vi "NegativeImage.vi"(11 "Picture in":picture) -> (3 "New Picture out":picture)   [LabVIEW 2023]
doc: "This VI creates a negative of the input picture. \n\nPicture in - picture input.\nNew Picture out - a negative picture input."
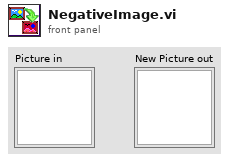
[diagram p1: front panel]
types:
  T1 = typedef "imagedata.ctl" = cluster{"image type":i32, "image depth":i32, "image":u8[], "mask":u8[], "colors":u32[], "Rectangle":cluster{"left":i16, "top":i16, "right":i16, "bottom":i16}}
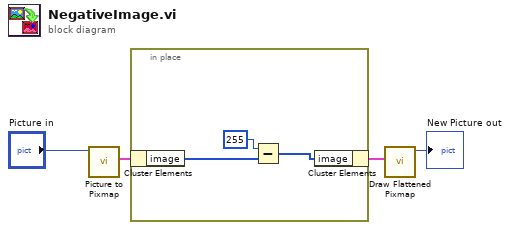
[diagram p0: block diagram]
diagram:
  n1 = call <vilib>:"Picture to Pixmap.vi"("picture"="Picture in") -> ("image data"=w2:T1)  [unwired: 9 in, 1 out]
  n2 = in-place "In Place Element Structure" {
    n3 = in-place-cluster #1(w2) -> ("image"=w7:u8[])
    n4 = Subtract(x=255, y=w7) -> (x-y=w6:i32[])
    n5 = in-place-cluster #1("image"=w6) -> (w1:T1)
  }
  n6 = call <vilib>:"Draw Flattened Pixmap.vi"("image data"=w1) -> ("new picture"=→"New Picture out":picture)  [unwired: 8 in]
